vi "Write clImpairConfig.vi"(8 "error in (no error)":errorcluster, 10 "clImpairConfig":T1={"FilterType"="", "bPosSeq"=TRUE}, 11 "PmuImpairPluginBase in":refnum<class "PmuImpairPluginBase.lvclass">) -> (0 "error out":errorcluster, 3 "PmuImpairPluginBase out":refnum<class "PmuImpairPluginBase.lvclass">)   [LabVIEW 2014, in "PmuImpairPlugins.lvlib" / "PmuImpairPluginBase.lvclass"]
uses:
  PmuImpairPluginBase.lvclass
  TypeDefs/clImpairConfig.ctl
  PmuImpairPluginBase.lvclass/PmuImpairPluginBase.ctl
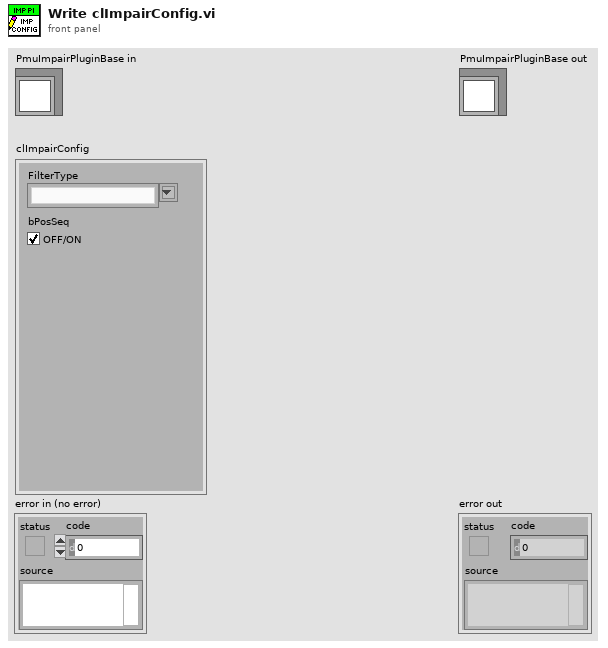
[diagram p1: front panel]
types:
  T1 = typedef "PmuImpairPlugins.lvlib/PmuImpairPluginBase.lvclass/clImpairConfig.ctl" = cluster{"FilterType":string, "bPosSeq":bool}
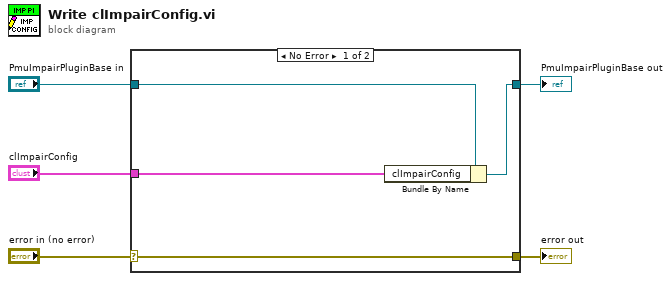
[diagram p0: block diagram]
diagram:
  n1 = case shown="No Error" "error in (no error)" {
    selector: "error in (no error)" -> [w9 w10]
    tunnel: [w9 w10] -> w4
    tunnel: [w7 w11] -> w2
    tunnel: "PmuImpairPluginBase in" -> [w8 w11]
    tunnel: "clImpairConfig" -> [w6 _]
    frame No Error {
      n2 = Bundle By Name(cluster=w8, "clImpairConfig"=w6) -> (w7:refnum<class "PmuImpairPluginBase.lvclass">)
    }
    frame Error {
    }
  }
  "error out" <- w4
  "PmuImpairPluginBase out" <- w2
